vi "Equalization.vi"(0 "connection ID":refnum<k5>, 1 "Pixel Register":u32[](array[numeric])=[671965161, 384, 671965161, 384, 671965161, 384, 671965161, 384, 671965161, 384, 671965161, 384, 671965161, 384, 671965161, 384, 671965161, 384, 671965161, 384, 671965161, 384, 671965161, 384, 671965161, 384, 671965161, 384, 671965161, 384, 671965161, 384, 671965161, 384, 671965161, 384, 671965161, 384, 671965161, 384, 671965161, 384, 671965161, 384, 671965161, 384, 671965161, 384, 671965161, 384, 671965161, 384, 671965161, 384, 671965161, 384, 671965161, 384, 671965161, 384, 671965161, 384, 671965161, 384, 671965161, 384, 671965161, 384, 671965161, 384, 671965161, 384, 671965161, 384, 671965161, 384, 671965161, 384, 671965161, 384, 671965161, 384, 671965161, 384, 671965161, 384, 671965161, 384, 671965161, 384, 671965161, 384, 671965161, 384, 671965161, 384, 671965161, 384, 671965161, 384, 671965161, 384, 671965161, 384, 671965161, 384, 671965161, 384, 671965161, 384, 671965161, 384, 671965161, 384, 671965161, 384, 671965161, 384, 671965161, 384, 671965161, 384, 671965161, 384, 671965161, 384, 671965161, 384, 671965161, 384, 671965161, 384, 671965161, 384, 671965161, 384, 671965161, 384, 671965161, 384, 671965161, 384, 671965161, 384, 671965161, 384, 671965161, 384, 671965161, 384, 671965161, 384, 671965161, 384, 671965161, 384, 671965161, 384, 671965161, 384, 671965161, 384, 671965161, 384, 671965161, 384, 671965161, 384, 671965161, 384, 671965161, 384, 671965161, 384, 671965161, 384, 671965161, 384, 671965161, 384, 671965161, 384, 671965161, 384, 671965161, 384, 671965161, 384, 671965161, 384, 671965161, 384, 671965161, 384, 671965161, 384, 671965161, 384, 671965161, 384] format="%x", 2 "Global Register":u32[](array[numeric])=[68228136, 235670329, 4294967264, 4294967295, 4294967295, 511] format="%x", 3 "Equalization parameters":u32[](array[numeric])=[240000, 5, 1600, 900, 100, 4400000, 400000, 2, 0, 99, 2, 40000, 38, 0], 4 "Equalization timeout":u32=2250000000 format="%x", 5 "error in (no error)":errorcluster, 6 "ChipID":u32=65535 format="%x", 8 "LayerID":u32=65535 format="%x") -> (13 "Answer":string, 14 "connection ID out":refnum<k5>, 16 "EQ Data and Report":u32[](array[numeric]) format="%x", 17 "EQ time (s)":u32, 18 "EQ Timeout":bool, 19 "error out":errorcluster)   [LabVIEW 2015, in "VIPM2.lvlib"]
uses:
  VIPM2.lvlib
panel:
  out "Ready to receive parameters":string
  # "Equalization"
  # "If red = timeout"
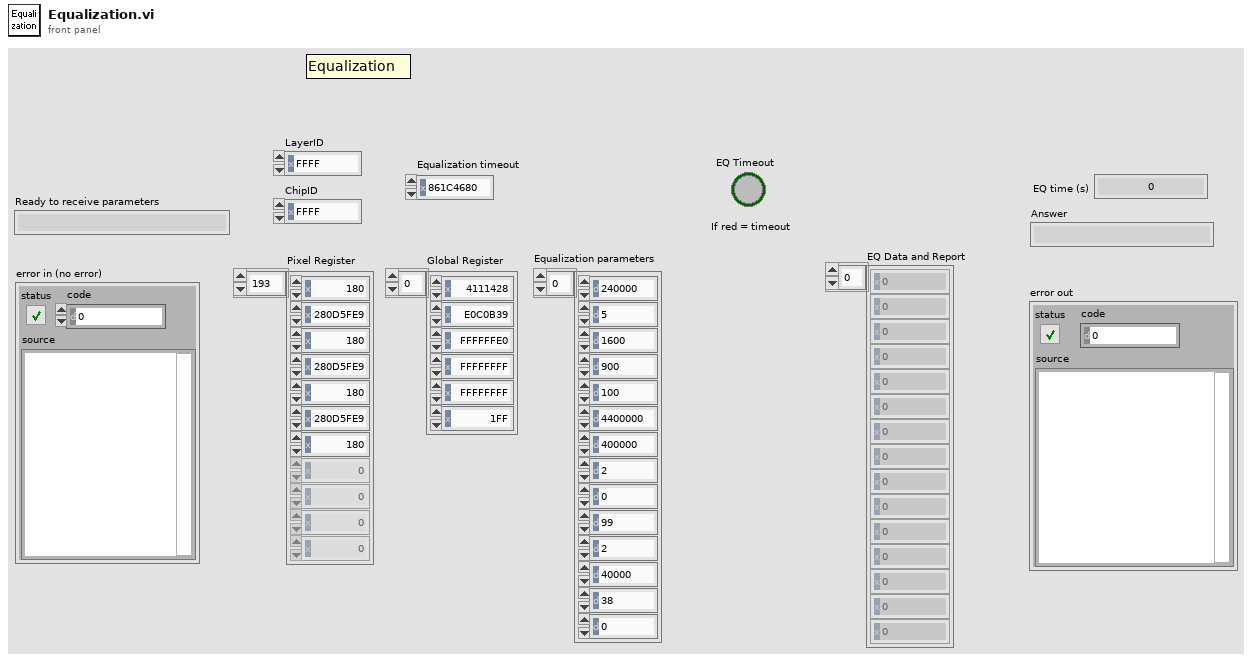
[diagram p1: front panel]
types:
  T1 = enum16{"Standard", "Buffered", "CRLF", "Immediate"}
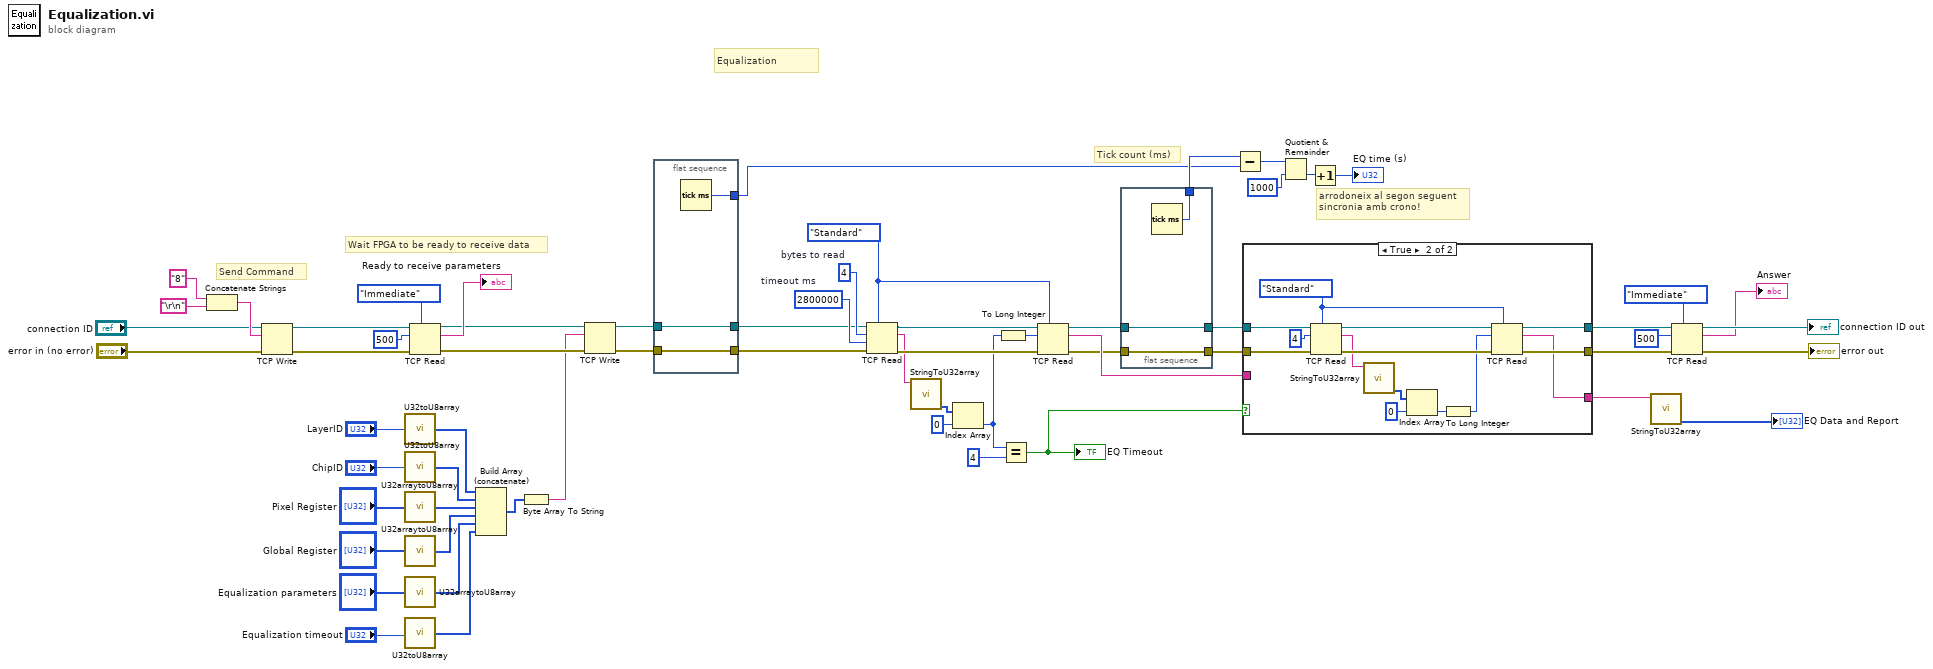
[diagram p0: block diagram]
diagram:
  w23 = 2800000  # timeout ms
  w35 = 4  # bytes to read
  w36 = T1."Standard" ("mode (standard)")
  # "arrodoneix al segon seguent\nsincronia amb crono!"
  # "Tick count (ms)"
  # "Wait FPGA to be ready to receive data"
  # "Send Command"
  # "Equalization"
  n1 = Concatenate Strings("8" ("string"), "\r\n") -> (w60:string)
  n2 = TCP Write(connection ID="connection ID", data in=w60, error in (no error)="error in (no error)") -> (connection ID out=w54:refnum<k5>, error out=w53:errorcluster)  [unwired: 1 in, 1 out]
  n3 = call "U32toU8array.vi"("x"="LayerID") -> ("ArrayU8"=w42:u8[])
  n4 = call "U32toU8array.vi"("x"="ChipID") -> ("ArrayU8"=w40:u8[])
  n5 = call "U32arraytoU8array.vi"("ArrayU32"="Pixel Register") -> ("ArrayU8"=w31:u8[])
  n6 = call "U32arraytoU8array.vi"("ArrayU32"="Global Register") -> ("ArrayU8"=w28:u8[])
  n7 = call "U32arraytoU8array.vi"("ArrayU32"="Equalization parameters") -> ("ArrayU8"=w26:u8[])
  n8 = call "U32toU8array.vi"("x"="Equalization timeout") -> ("ArrayU8"=w24:u8[])
  n9 = TCP Read(connection ID=w54, bytes to read=500, error in (no error)=w53, 7:T1."Immediate" ("mode (standard)")) -> (connection ID out=w51:refnum<k5>, data out=→"Ready to receive parameters":string, error out=w50:errorcluster)  [unwired: 1 in]
  n10 = Build Array (concatenate)(w42, w40, w31, w28, w26, w24) -> (w43:u8[])
  n11 = Byte Array To String(unsigned byte array=w43) -> (string=w49:string)
  n12 = TCP Write(connection ID=w51, data in=w49, error in (no error)=w50) -> (connection ID out=w14:refnum<k5>, error out=w17:errorcluster)  [unwired: 1 in, 1 out]
  n13 = flat-sequence {
    tunnel: w17 -> [w65]
    tunnel: [w65] -> w16
    tunnel: [w64] -> w15
    tunnel: w14 -> [w64]
    tunnel: [w63] -> w8
    frame #0 {
      n14 = Tick Count (ms)() -> (millisecond timer value=w63:u32)
    }
  }
  n15 = TCP Read(connection ID=w15, bytes to read=w35, error in (no error)=w16, 7:w36, 9:w23) -> (connection ID out=w39:refnum<k5>, data out=w34:string, error out=w38:errorcluster)
  n16 = call "StringToU32array.vi"("String"=w34) -> ("U32array"=w33:u32[])  [unwired: 2 out]
  n17 = Index Array(array=w33, index=0) -> (element=w2:u32)
  n18 = To Long Integer(number=w2) -> (32bit integer=w3:i32)
  n19 = Equal?(x=w2, y=u32 4) -> (x = y?=w21:bool)
  "EQ Timeout" <- w21
  n20 = TCP Read(connection ID=w39, bytes to read=w3, error in (no error)=w38, 7:w36) -> (connection ID out=w10:refnum<k5>, data out=w20:string, error out=w13:errorcluster)  [unwired: 1 in]
  n21 = flat-sequence {
    tunnel: w13 -> [w68]
    tunnel: [w68] -> w12
    tunnel: [w67] -> w11
    tunnel: w10 -> [w67]
    tunnel: [w66] -> w9
    frame #0 {
      n22 = Tick Count (ms)() -> (millisecond timer value=w66:u32)
    }
  }
  n23 = Subtract(x=w9, y=w8) -> (x-y=w6:u32)
  n24 = case shown="True" w21 {
    tunnel: w11 -> [w70 w83]
    tunnel: w12 -> [w71 w82]
    tunnel: [w71 w80] -> w18
    tunnel: w20 -> [w69 _]
    tunnel: [w70 w75] -> w19
    tunnel: [w69 w72] -> w1
    frame False {
    }
    frame True {
      w84 = T1."Standard" ("mode (standard)")
      n25 = TCP Read(connection ID=w83, bytes to read=4, error in (no error)=w82, 7:w84) -> (connection ID out=w79:refnum<k5>, data out=w77:string, error out=w81:errorcluster)  [unwired: 1 in]
      n26 = call "StringToU32array.vi"("String"=w77) -> ("U32array"=w76:u32[])  [unwired: 2 out]
      n27 = Index Array(array=w76, index=0) -> (element=w74:u32)
      n28 = To Long Integer(number=w74) -> (32bit integer=w73:i32)
      n29 = TCP Read(connection ID=w79, bytes to read=w73, error in (no error)=w81, 7:w84) -> (connection ID out=w75:refnum<k5>, data out=w72:string, error out=w80:errorcluster)  [unwired: 1 in]
    }
  }
  n30 = Quotient & Remainder(x=w6, y=u32 1000) -> (floor(x/y)=w5:u32)  [unwired: 1 out]
  n31 = Increment(x=w5) -> (x+1=→"EQ time (s)":u32)
  n32 = call "StringToU32array.vi"("String"=w1) -> ("U32array"=→"EQ Data and Report":u32[])  [unwired: 2 out]
  n33 = TCP Read(connection ID=w19, bytes to read=500, error in (no error)=w18, 7:T1."Immediate" ("mode (standard)")) -> (connection ID out=→"connection ID out":refnum<k5>, data out=→"Answer":string, error out=→"error out":errorcluster)  [unwired: 1 in]
